vi "Build Low Priority Check.vi"(6 "Group":i32, 7 "Virtual Memory Unit in":refnum<class "Virtual Memory Unit.lvclass">, 8 "error in (no error)":errorcluster, 10 "Starting Address":u16 format="%04x", 11 "Major Frame in":refnum<class "Major Frame.lvclass">) -> (0 "error out":errorcluster, 2 "Next Available Address":u16 format="%04x", 3 "Major Frame out":refnum<class "Major Frame.lvclass">, 5 "Virtual Memory Unit out":refnum<class "Virtual Memory Unit.lvclass">)   [LabVIEW 2020, in "BCI-1553 API.lvlib" / "Major Frame.lvclass"]
doc: "Builds a asynchronous low priority check instruction set.\n\nThis command set is triggerable by GP5, GP6, or GP7, depending on the group.\n\nGroup 0: GP5\nGroup 1: GP6\nGroup 2: GP7"
uses:
  Major Frame.lvclass
  Dependencies/Virtual Memory Unit/Virtual Memory Unit.lvclass
  TypeDefs/BC Op Codes - Verbose.ctl
  TypeDefs/BC Condition Codes.ctl
  Major Frame.lvclass/Major Frame.ctl
  BCI-1553 API.lvlib
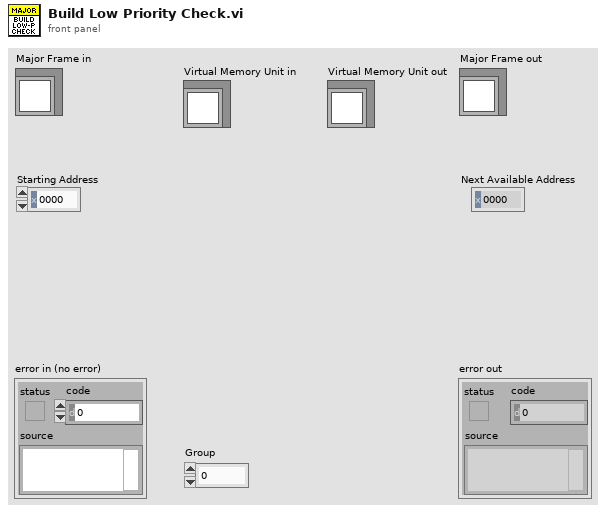
[diagram p1: front panel]
types:
  T1 = typedef "BCI-1553 API.lvlib/BC Condition Codes.ctl" = enum16{"GP0 == 1 || LT", "GP1 == 1 || NE", "GP2 == 1", "GP3 == 1", "GP4 == 1", "GP5 == 1", "GP6 == 1", "GP7 == 1", "NORESP", "FMTERR", "GOODBLOCK", "MSKSTATSET", "BADMSG", "1RETRY", "2RETRY", "ALWAYS"}
  T2 = typedef "BCI-1553 API.lvlib/BC Op Codes - Verbose.ctl" = enum16{"EXECUTE MSG", "EXECUTE MSG GO", "JUMP", "CALL SUBROUTINE", "RETURN", "INTERRUPT REQUEST", "HALT", "DELAY", "WAIT FRAME TIMER = 0", "COMPARE FRAME TIMER", "COMPARE MSG TIMER", "LOAD TIME TAG CTR", "LOAD TIME TAG CTR HI", "LOAD FRAME TIMER", "START FRAME TIMER", "PUSH TIME TAG COUNT", "PUSH TIME TAG COUNT HI", "PUSH TIME TAG COUNT BOTH", "PUSH BLOCK STATUS WORD", "PUSH CURRENT VALUE", "PUSH INDIRECT", "WAIT EXT TRIGGER", "EXECUTE AND FLIP", "EXECUTE, FLIP, GO", "WRITE VALUE TO WMI", "WRITE VALUE TO MEM", "DECREMENT RAM, SKIP", "FLAG"}
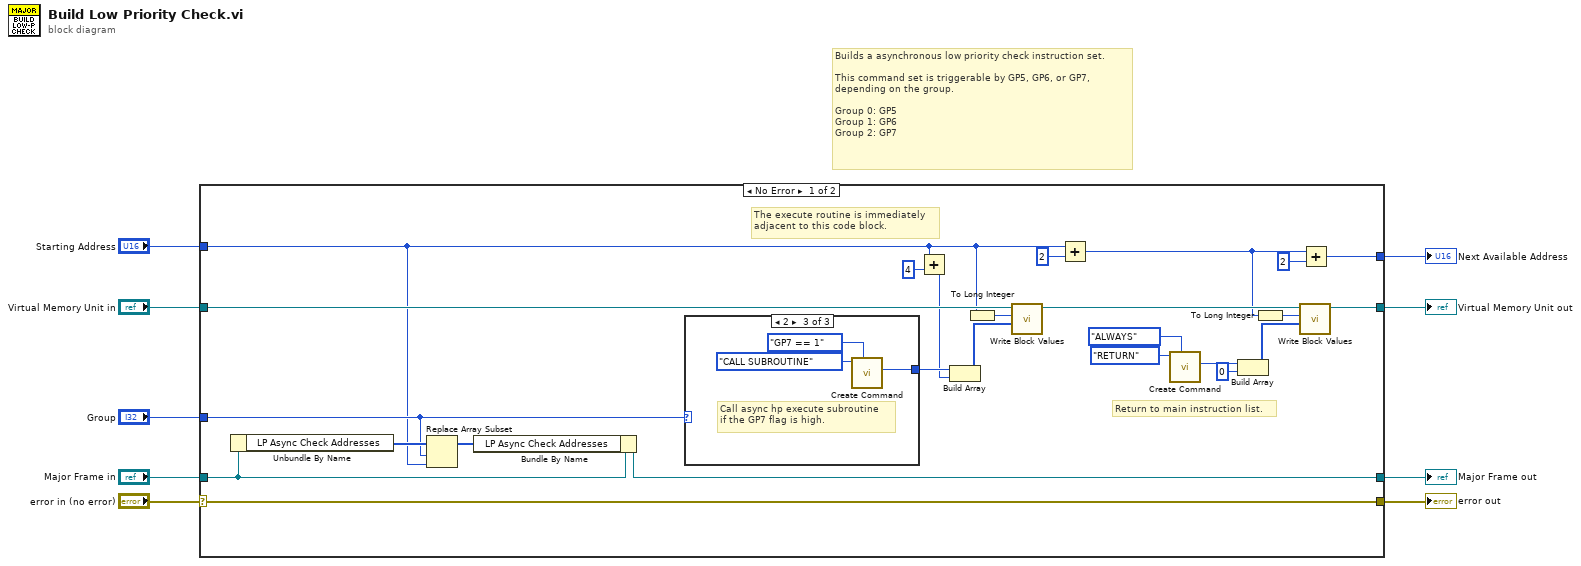
[diagram p0: block diagram]
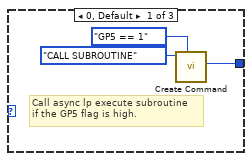
[diagram p2: hidden frame]
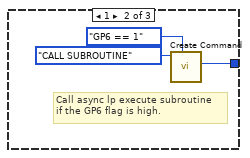
[diagram p3: hidden frame]
diagram:
  # "Builds a asynchronous low priority check instruction set.\n\nThis command set is triggerable by GP5, GP6, or GP7,\ndepending on the group.\n\nGroup 0: GP5\nGroup 1: GP6\nGroup 2: GP7"
  n1 = case shown="No Error" "error in (no error)" {
    selector: "error in (no error)" -> [w34 w45]
    tunnel: [w34 w45] -> w4
    tunnel: [w12 w44] -> w3
    tunnel: "Major Frame in" -> [w13 w44]
    tunnel: "Virtual Memory Unit in" -> [w33 _]
    tunnel: [w21 _] -> w2
    tunnel: "Starting Address" -> [w10 _]
    tunnel: "Group" -> [w11 _]
    tunnel: [w16 _] -> w1
    frame No Error {
      # "Return to main instruction list."
      # "The execute routine is immediately\nadjacent to this code block."
      n2 = Unbundle By Name(w13) -> ("LP Async Check Addresses"=w15:u16[])
      n3 = Replace Array Subset(array=w15, new element=w10, index=w11) -> (w14:u16[])
      n4 = Bundle By Name(cluster=w13, "LP Async Check Addresses"=w14) -> (w12:refnum<class "Major Frame.lvclass">)
      n5 = case shown="2" w11 {
        tunnel: [w35 w38 w41] -> w32
        frame 0, Default {
          # "Call async lp execute subroutine\nif the GP5 flag is high."
          n6 = call "Create Command.vi"("Condition"=BC_Condition_Codes."GP5 == 1", "Op Code"=BC_Op_Codes_-_Verbose."CALL SUBROUTINE") -> ("Instruction"=w35:u16)  [unwired: 8 in, 1 out]
        }
        frame 1 {
          # "Call async lp execute subroutine\nif the GP6 flag is high."
          n7 = call "Create Command.vi"("Condition"=BC_Condition_Codes."GP6 == 1", "Op Code"=BC_Op_Codes_-_Verbose."CALL SUBROUTINE") -> ("Instruction"=w38:u16)  [unwired: 8 in, 1 out]
        }
        frame 2 {
          # "Call async hp execute subroutine\nif the GP7 flag is high."
          n8 = call "Create Command.vi"("Condition"=BC_Condition_Codes."GP7 == 1", "Op Code"=BC_Op_Codes_-_Verbose."CALL SUBROUTINE") -> ("Instruction"=w41:u16)  [unwired: 8 in, 1 out]
        }
      }
      n9 = Add(x=w10, y=u16 4 ("x")) -> (x+y=w31:u16)
      n10 = Build Array(w32, w31) -> (w29:u16[])
      n11 = To Long Integer(number=w10) -> (32bit integer=w28:i32)
      n12 = call "Write Block Values.vi"("Write Block"=w29, "Start Index"=w28, "Virtual Memory Unit in"=w33) -> ("Virtual Memory Unit out"=w22:refnum<class "Virtual Memory Unit.lvclass">)  [unwired: 7 in, 1 out]
      n13 = Add(x=w10, y=u16 2) -> (x+y=w17:u16)
      n14 = call "Create Command.vi"("Condition"=BC_Condition_Codes."ALWAYS", "Op Code"=BC_Op_Codes_-_Verbose."RETURN") -> ("Instruction"=w20:u16)  [unwired: 8 in, 1 out]
      n15 = Build Array(w20, u16 0 ("element")) -> (w24:u16[])
      n16 = To Long Integer(number=w17) -> (32bit integer=w23:i32)
      n17 = call "Write Block Values.vi"("Write Block"=w24, "Start Index"=w23, "Virtual Memory Unit in"=w22) -> ("Virtual Memory Unit out"=w21:refnum<class "Virtual Memory Unit.lvclass">)  [unwired: 7 in, 1 out]
      n18 = Add(x=w17, y=u16 2) -> (x+y=w16:u16)
    }
    frame Error {
    }
  }
  "error out" <- w4
  "Major Frame out" <- w3
  "Virtual Memory Unit out" <- w2
  "Next Available Address" <- w1
